vi "dynamic mapping.vi"(8 "error in":errorcluster, 10 "channels available":refnum<class "TBM channel.lvclass">[](array[class]), 11 "module configuration in":refnum<class "TDMS datalogger configuration.lvclass">) -> (0 "error out":errorcluster, 2 "reservations":T1[](array[typedef]), 3 "module configuration out":refnum<class "TDMS datalogger configuration.lvclass">)   [LabVIEW 2015, in "TDMS datalogger configuration.lvclass"]
doc: "Provides an interface for dynamically mapping data at runtime instead of static mapping. For example, a module may which to log all data in a given execution system to disk. In this case, it would register to read data from all groups defined as inputs to the system. Calling code is responsible for providing this data to the requesting component. There is no way to \"undo\" reservations within a component without directly manipulating the component's data."
uses:
  TDMS datalogger configuration.lvclass
  <vilib>/NI/Tag Bus Module Framework/channel/TBM channel.lvclass
  <vilib>/NI/Tag Bus Module Framework/module configuration/channel reservation.ctl
  TDMS datalogger configuration.lvclass/TDMS datalogger configuration.ctl
  <vilib>/NI/Tag Bus/tag/tag descriptor.lvclass/tag descriptor.ctl
  <vilib>/NI/Tag Bus Module Framework/channel/channel classification.ctl
  <vilib>/NI/Tag Bus Module Framework/channel/TBM channel.lvclass/TBM channel.ctl
  <vilib>/NI/Tag Bus Module Framework/channel/Write channel classification.vi
  Read channel pattern matches.vi
  <vilib>/NI/Tag Bus/tag/read data type.vi
  <vilib>/NI/Tag Bus/tag/read tag name.vi
  <vilib>/NI/Tag Bus/tag/tag descriptor.lvclass
  <vilib>/NI/Tag Bus Module Framework/module configuration/TBM module configuration.lvclass
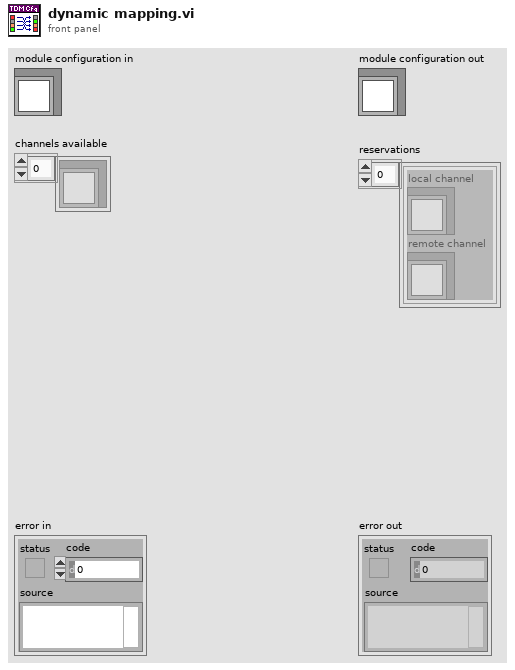
[diagram p1: front panel]
types:
  T1 = typedef "TBM module configuration.lvclass/channel reservation.ctl" = cluster{"local channel":refnum<class "TBM channel.lvclass">, "remote channel":refnum<class "TBM channel.lvclass">}
  T2 = typedef "tag bus.lvlib/tag descriptor.lvclass/Data Type.ctl" = enum16{"Double", "Single", "I64", "I32", "I16", "I8", "U64", "U32", "U16", "U8", "Boolean", "String", "Array of Double", "Array of Single", "Array of I64", "Array of I32", "Array of I16", "Array of I8", "Array of U64", "Array of U32", "Array of U16", "Array of U8", "Array of Boolean", "Array of String"}
  T3 = typedef "TBM channel.lvclass/channel classification.ctl" = enum16{"input data", "output data", "processing parameter", "processing result"}
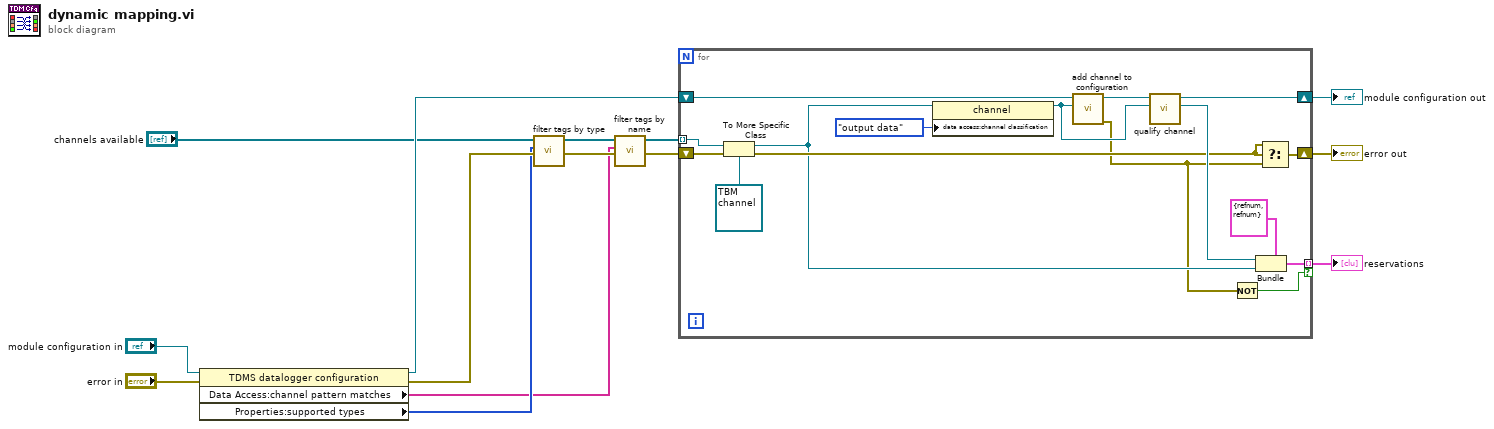
[diagram p0: block diagram]
diagram:
  n1 = property class="TDMS datalogger configuration"(reference="module configuration in", error in="error in") -> (reference out=w10:refnum<class "TDMS datalogger configuration.lvclass">, error out=w8:errorcluster, "Data Access:channel pattern matches"=w2:string[], "Properties:supported types"=w4:T2[])
  n2 = call <vilib>:"filter tags by type.vi"("allowable types"=w4, "tags in"="channels available") -> ("filtered tags"=w3:refnum<class "tag descriptor.lvclass">[])  [unwired: 9 in]
  n3 = call <vilib>:"filter tags by name.vi"("allowable patterns"=w2, "tags in"=w3) -> ("filtered tags"=w1:refnum<class "tag descriptor.lvclass">[])  [unwired: 9 in]
  n4 = for {
    shift-right: [w26] -> w9
    shift-left: w10 -> [w28]
    tunnel: w1 -> [w16] mode=indexing
    shift-right: [w22] -> w7
    shift-left: w8 -> [w23]
    tunnel: [w21] -> w6 mode=indexing if=w20
    n5 = To More Specific Class(target class=refnum<class "TBM channel.lvclass"> refnum ("channel"), reference=w16, error in=w23) -> (specific class reference=w14:refnum<class "TBM channel.lvclass">, error out=w17:errorcluster)
    n6 = property class="channel"(reference=w14, "data access:channel classification"=channel_classification."output data" ("channel classification")) -> (reference out=w18:refnum<class "TBM channel.lvclass">)  [unwired: 1 in, 1 out]
    n7 = call "add channel to configuration.vi"("TBM channel in"=w18, "TDMS datalogger configuration in"=w28) -> ("error out"=w13:errorcluster, "TDMS datalogger configuration out"=w27:refnum<class "TDMS datalogger configuration.lvclass">)  [unwired: 8 in]
    n8 = call <vilib>:"qualify channel.vi"("unqualified channel"=w18, "module configuration in"=w27) -> ("qualified channel"=w24:refnum<class "TBM channel.lvclass">, "module configuration out"=w26:refnum<class "TDMS datalogger configuration.lvclass">)  [unwired: 8 in]
    n9 = Not(x=w13) -> (.not. x?=w20:bool)
    n10 = Bundle(cluster=T1 {"local channel"=refnum, "remote channel"=refnum} ("reservation"), "local channel"=w24, "remote channel"=w14) -> (w21:T1)
    n11 = Select(t=w17, s=w17, f=w13) -> (s? t:f=w22:errorcluster)
  }
  "error out" <- w7
  "module configuration out" <- w9
  "reservations" <- w6
